vi "pf Get Camera Property I.vi"(8 "error in (no error)":errorcluster, 10 "pProperty":string, 11 "iPort":i32) -> (0 "error out":errorcluster, 3 "function return":u32)   [LabVIEW 2025, in "Photonfocus_Toolkit.lvlib"]
doc: "PFCONFIG_API int pfGetCameraPropertyI(const char* pProperty);"
uses:
  Photonfocus_Toolkit.lvlib
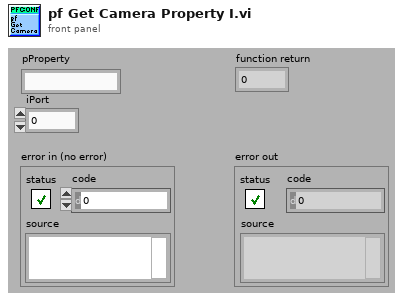
[diagram p1: front panel]
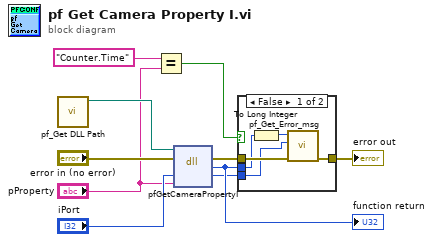
[diagram p0: block diagram]
diagram:
  n1 = call "pf_Get DLL Path.vi"() -> ("DLL path"=w9:path)  [unwired: 1 in, 10 out]
  n2 = Equal?(x="Counter.Time", y="pProperty") -> (x = y?=w2:bool)
  n3 = dll-call lib="S:/Progetti/Photonfocus/Codice/DEV/PFConfig_lvlib/PFConfig.*" fn="pfGetCameraPropertyI"(path in=w9, error in="error in (no error)", "iPort"="iPort", "pProperty"="pProperty") -> (error out=w8:errorcluster, "return type"=w6:u32, "iPort"=w1:i32)  [unwired: 2 in, 1 out]
  "function return" <- w6
  n4 = case shown="False" w2 {
    tunnel: w8 -> [w15 w16]
    tunnel: [w14 w16] -> w7
    tunnel: w6 -> [w12 _]
    tunnel: w1 -> [w11 _]
    frame False {
      n5 = To Long Integer(number=w12) -> (32bit integer=w13:i32)
      n6 = call "pf_Get_Error_msg.vi"("error in (no error)"=w15, "iPort"=w11, "error code"=w13) -> ("error out"=w14:errorcluster)  [unwired: 8 out]
    }
    frame True {
    }
  }
  "error out" <- w7
